vi "subVI_FitLorentzien.vi"(5 "Background Spec":dbl[](array[numeric]), 6 "X":dbl[](array[numeric]), 7 "Y":dbl[](array[numeric])) -> (0 "XY Graph":cluster{"X":dbl[], "best nonlinear fit":dbl[]}[](graph) caption="Width 2.000 meV", 1 "residue":dbl, 2 "best fit parameters":dbl[](array[numeric]), 3 "best nonlinear fit":dbl[](array[numeric]))   [LabVIEW 2019]
uses:
  <vilib>/gmath/NumericalOptimization/Nonlinear Curve Fit LM formula string.vi
  <vilib>/gmath/NI_Gmath.lvlib
panel:
  in  "Stop":bool
  in  "termination":cluster{"max iteration":i32, "tolerance":dbl}={"max iteration"=400, "tolerance"=1e-08}
  in  "Test?":bool
  in  "Start Params a, x0, FWHM":dbl[](array[numeric])
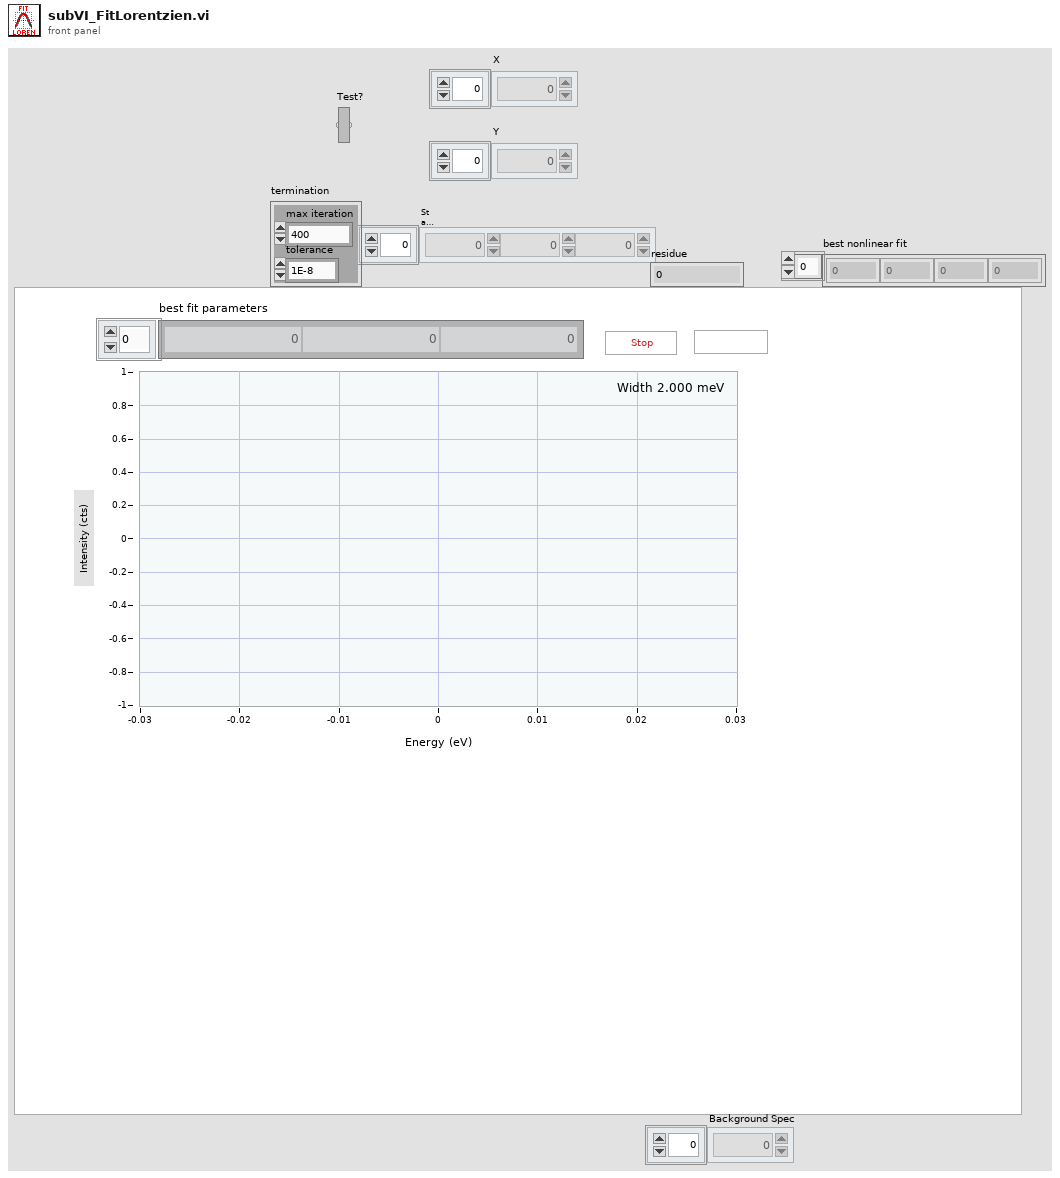
[diagram p1: front panel]
types:
  T1 = cluster{"model":string, "Parameters":string[], "x":string}
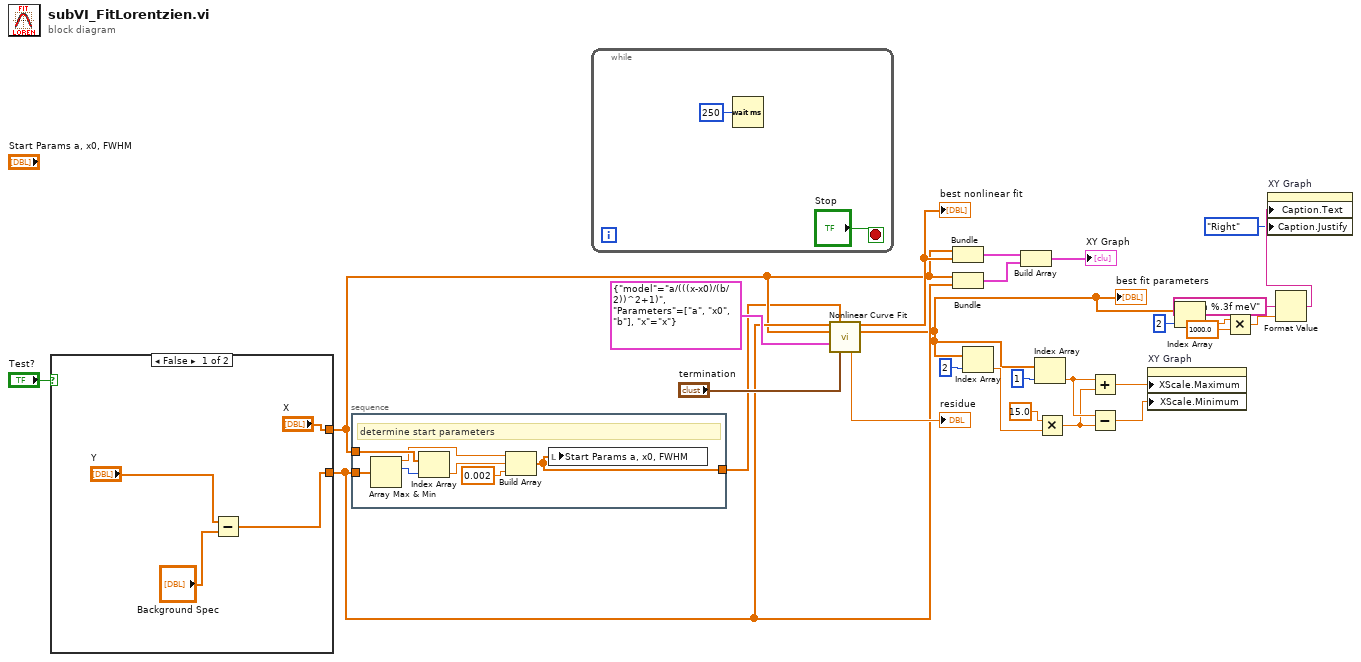
[diagram p0: block diagram]
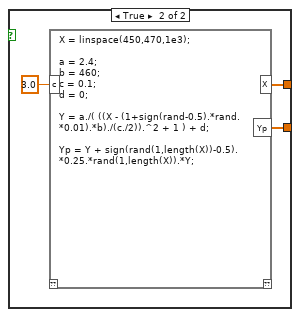
[diagram p2: hidden frame]
diagram:
  n1 = case shown="False" "Test?" {
    tunnel: ["X" w33] -> w10
    tunnel: [w29 w32] -> w11
    frame False {
      n2 = Subtract(x="Y", y="Background Spec") -> (x-y=w29:dbl[])
    }
    frame True {
      n3 = script code="X = linspace(450,470,1e3);\n\na = 2.4;\nb = 460;\nc = 0.1;\nd = 0;\n\nY = a./( ((X - (1+sign(rand-0.5).*rand.*0.01).*b)./(c./2)).^2 + 1 ) + d;\n\nYp = Y + sign(rand(1,length(X))-0.5).*0.25.*rand(1,length(X)).*Y;"("c"=3.0 ("Real")) -> ("Yp"=w32:dbl[], "X"=w33:dbl[])  [unwired: 1 in, 1 out]
    }
  }
  n4 = stacked-sequence {
    tunnel: w11 -> [w41]
    tunnel: w10 -> [w39]
    tunnel: [w35] -> w9
    frame #0 {
      # "determine start parameters"
      n5 = Array Max & Min(array=w41) -> (max value=w38:dbl, max index (indices)=w40:i32)  [unwired: 2 out]
      n6 = Index Array(array=w39, index=w40) -> (element=w37:dbl)
      n7 = Build Array(w38, w37, 0.002 ("element")) -> (w35:dbl[])
      n8 = local write "Start Params a, x0, FWHM"(w35) -> ()
    }
  }
  n9 = while {
    stop <- "Stop" stop-if-true
    n10 = Wait (ms)(milliseconds to wait=u32 250) -> ()  [unwired: 1 out]
  }
  n11 = call-poly <vilib>:"Nonlinear Curve Fit.vi"("Y"=w11, "initial parameters"=w9, "X"=w10, "model description"=T1 {"model"="a/(((x-x0)/(b/2))^2+1)", "Parameters"=["a", "x0", "b"], "x"="x"}, "termination"="termination") -> ("best nonlinear fit"=w23:dbl[], "best fit parameters"=w8:dbl[], "residue"=→"residue":dbl)  [unwired: 6 in, 2 out]
  "best fit parameters" <- w8
  "best nonlinear fit" <- w23
  n12 = Bundle("X"=w10, "best nonlinear fit"=w23) -> (w14:cluster{"X":dbl[], "best nonlinear fit":dbl[]})  [unwired: 1 in]
  n13 = Bundle("X"=w10, w11) -> (w13:cluster{"X":dbl[], dbl[]})  [unwired: 1 in]
  n14 = Index Array(array=w8, index=2) -> (element=w19:dbl)
  n15 = Build Array(w14, w13) -> (→"XY Graph":cluster{"X":dbl[], "best nonlinear fit":dbl[]}[])
  n16 = Index Array(array=w8, index=1) -> (element=w18:dbl)
  n17 = Multiply(x=15.0, y=w19) -> (x*y=w17:dbl)
  n18 = Add(x=w18, y=w17) -> (x+y=w15:dbl)
  n19 = Subtract(x=w18, y=w17) -> (x-y=w16:dbl)
  n20 = property on="XY Graph" class="XYGraph (strict)"("XScale.Maximum"=w15, "XScale.Minimum"=w16) -> ()  [unwired: 2 in, 2 out]
  n21 = Index Array(array=w8, index=2) -> (element=w6:dbl)
  n22 = Multiply(x=w6, y=1000.0) -> (x*y=w4:dbl)
  n23 = Format Value(format string="Width %.3f meV", value (0)=w4) -> (output string=w2:string)  [unwired: 1 in]
  n24 = property on="XY Graph" class="XYGraph (strict)"("Caption.Text"=w2, "Caption.Justify"=enum16{"Left", "Center", "Right"}."Right" ("Caption.Justification")) -> ()  [unwired: 2 in, 2 out]
